vi "Range Array.vi"(3 "# Values":dbl format="%#_13g", 4 "Step":dbl format="%#_13g", 5 "Stop":dbl format="%#_13g", 6 "Start":dbl format="%#_13g") -> (1 "Range":dbl[](array[numeric]))   [LabVIEW 2013]
doc: "Create an array with the range of numbers parameterized by either {Start, Stop, Steps} OR {Start, Stop, # Values}. The former takes precedence over the latter in the event that both Steps and # Values are != 0."
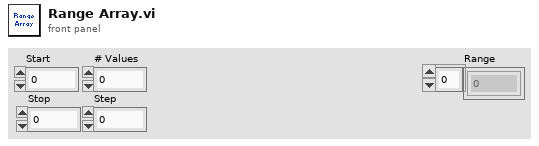
[diagram p1: front panel]
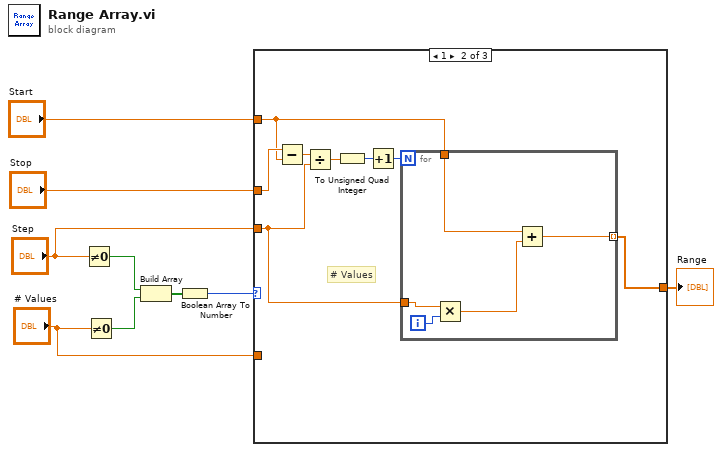
[diagram p0: block diagram]
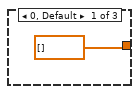
[diagram p2: hidden frame]
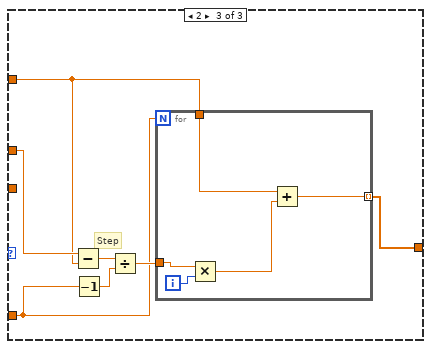
[diagram p3: hidden frame]
diagram:
  n1 = Not Equal To 0?(x="Step") -> (x != 0?=w9:bool)
  n2 = Not Equal To 0?(x="# Values") -> (x != 0?=w8:bool)
  n3 = Build Array(w9, w8) -> (w7:bool[])
  n4 = Boolean Array To Number(Boolean array=w7) -> (number=w6:u32)
  n5 = case shown="1" w6 {
    tunnel: [dbl[] [] w13 w24] -> w5
    tunnel: "Start" -> [_ w15 w28]
    tunnel: "Stop" -> [_ w18 w30]
    tunnel: "Step" -> [_ w14 _]
    tunnel: "# Values" -> [_ _ w25]
    frame 0, Default {
    }
    frame 1 {
      # "# Values"
      n6 = Subtract(x=w18, y=w15) -> (x-y=w17:dbl)
      n7 = Divide(x=w17, y=w14) -> (x/y=w16:dbl)
      n8 = To Unsigned Quad Integer(1:w16) -> (0:w11:u64)
      n9 = Increment(x=w11) -> (x+1=w12:u64)
      n10 = for {
        N: w12 -> [_]
        tunnel: w15 -> [w23]
        tunnel: w14 -> [w21]
        tunnel: [w19] -> w13 mode=indexing
        i -> [w22]
        n11 = Multiply(x=w21, y=w22) -> (x*y=w20:dbl)
        n12 = Add(x=w23, y=w20) -> (x+y=w19:dbl)
      }
    }
    frame 2 {
      # "Step"
      n13 = Subtract(x=w30, y=w28) -> (x-y=w29:dbl)
      n14 = Decrement(x=w25) -> (x-1=w26:dbl)
      n15 = Divide(x=w29, y=w26) -> (x/y=w27:dbl)
      n16 = for {
        N: w25 -> [_]
        tunnel: w28 -> [w35]
        tunnel: w27 -> [w33]
        tunnel: [w31] -> w24 mode=indexing
        i -> [w34]
        n17 = Multiply(x=w33, y=w34) -> (x*y=w32:dbl)
        n18 = Add(x=w35, y=w32) -> (x+y=w31:dbl)
      }
    }
  }
  "Range" <- w5
